vi "Set Constant Variables.vi"   [LabVIEW 2012]
uses:
  Robot Global Data.vi
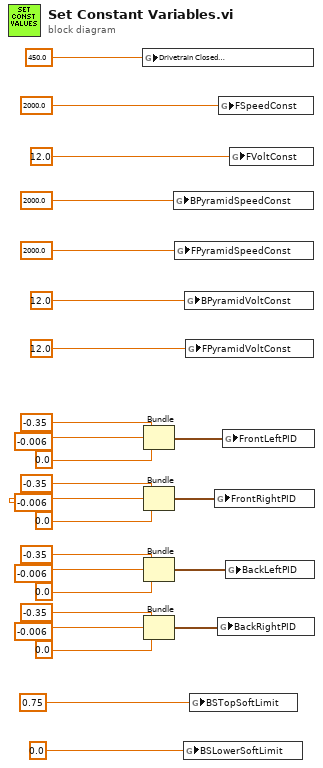
[diagram p0: block diagram]
diagram:
  n1 = global write "Robot Global Data.vi" "Drivetrain Closed\nLoop Max"(450.0 ("Drivetrain Closed\nLoop Max")) -> ()
  n2 = Bundle("P"=-0.35, "I"=-0.006, "D"=0.0) -> (w20:cluster{"P":dbl, "I":dbl, "D":dbl})  [unwired: 1 in]
  n3 = Bundle("P"=-0.35, "I"=-0.006, "D"=0.0) -> (w5:cluster{"P":dbl, "I":dbl, "D":dbl})  [unwired: 1 in]
  n4 = Bundle("P"=-0.35, "I"=-0.006, "D"=0.0) -> (w6:cluster{"P":dbl, "I":dbl, "D":dbl})  [unwired: 1 in]
  n5 = Bundle("P"=-0.35, "I"=-0.006, "D"=0.0) -> (w7:cluster{"P":dbl, "I":dbl, "D":dbl})  [unwired: 1 in]
  n6 = global write "Robot Global Data.vi" "BPyramidSpeedConst"(2000.0 ("FSpeedConst")) -> ()
  n7 = global write "Robot Global Data.vi" "FPyramidSpeedConst"(2000.0 ("FSpeedConst")) -> ()
  n8 = global write "Robot Global Data.vi" "BSLowerSoftLimit"(0.0 ("FVoltConst")) -> ()
  n9 = global write "Robot Global Data.vi" "BPyramidVoltConst"(12.0 ("FVoltConst")) -> ()
  n10 = global write "Robot Global Data.vi" "FPyramidVoltConst"(12.0 ("FVoltConst")) -> ()
  n11 = global write "Robot Global Data.vi" "BSTopSoftLimit"(0.75 ("FVoltConst")) -> ()
  n12 = global write "Robot Global Data.vi" "FrontRightPID"(w5) -> ()
  n13 = global write "Robot Global Data.vi" "BackRightPID"(w7) -> ()
  n14 = global write "Robot Global Data.vi" "FSpeedConst"(2000.0 ("FSpeedConst")) -> ()
  n15 = global write "Robot Global Data.vi" "FrontLeftPID"(w20) -> ()
  n16 = global write "Robot Global Data.vi" "BackLeftPID"(w6) -> ()
  n17 = global write "Robot Global Data.vi" "FVoltConst"(12.0 ("FVoltConst")) -> ()
